vi "ReviewQnsPaper1(SubVI).vi"(11 "connection reference":T2) -> (0 "close?":bool, 3 "connection reference out":T2)   [LabVIEW 2013]
uses:
  <vilib>/addons/database/Connection.llb/Conn ObjectReference.ctl
  FYP_LabviewGlobal(SubVI).vi
  <vilib>/addons/database/_DB Variant To Data/Database Variant To Data.xnode
  <vilib>/addons/database/NI_Database_API.lvlib
panel:
  out "Choice":string
  out "Answer":string
  out "D":bool
  out "C":bool
  out "B":bool
  out "A":bool
  out "D":string
  out "C":string
  out "B":string
  out "A":string
  out "DInd":bool
  out "CInd":bool
  out "BInd":bool
  out "AInd":bool
  out "Question":string
  out "Why?":string
  in  "SelectQn":T1(radio)
  in  "Close":bool
  out "Marks%":dbl
  out "TotalMarks":string
  # "% )"
  # "Your Score is :"
  # "("
  # "Questions:"
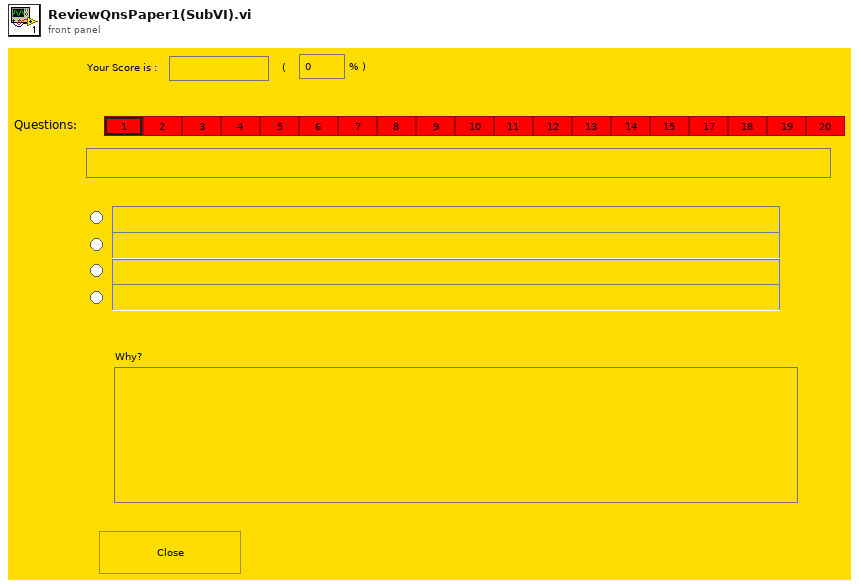
[diagram p1: front panel]
types:
  T1 = enum32{"1", "2", "3", "4", "5", "6", "7", "8", "9", "10", "11", "12", "13", "14", "15", "16", "17", "18", "19", "20"}
  T2 = typedef "NI_Database_API.lvlib/Conn ObjectReference.ctl" = refnum<k1>
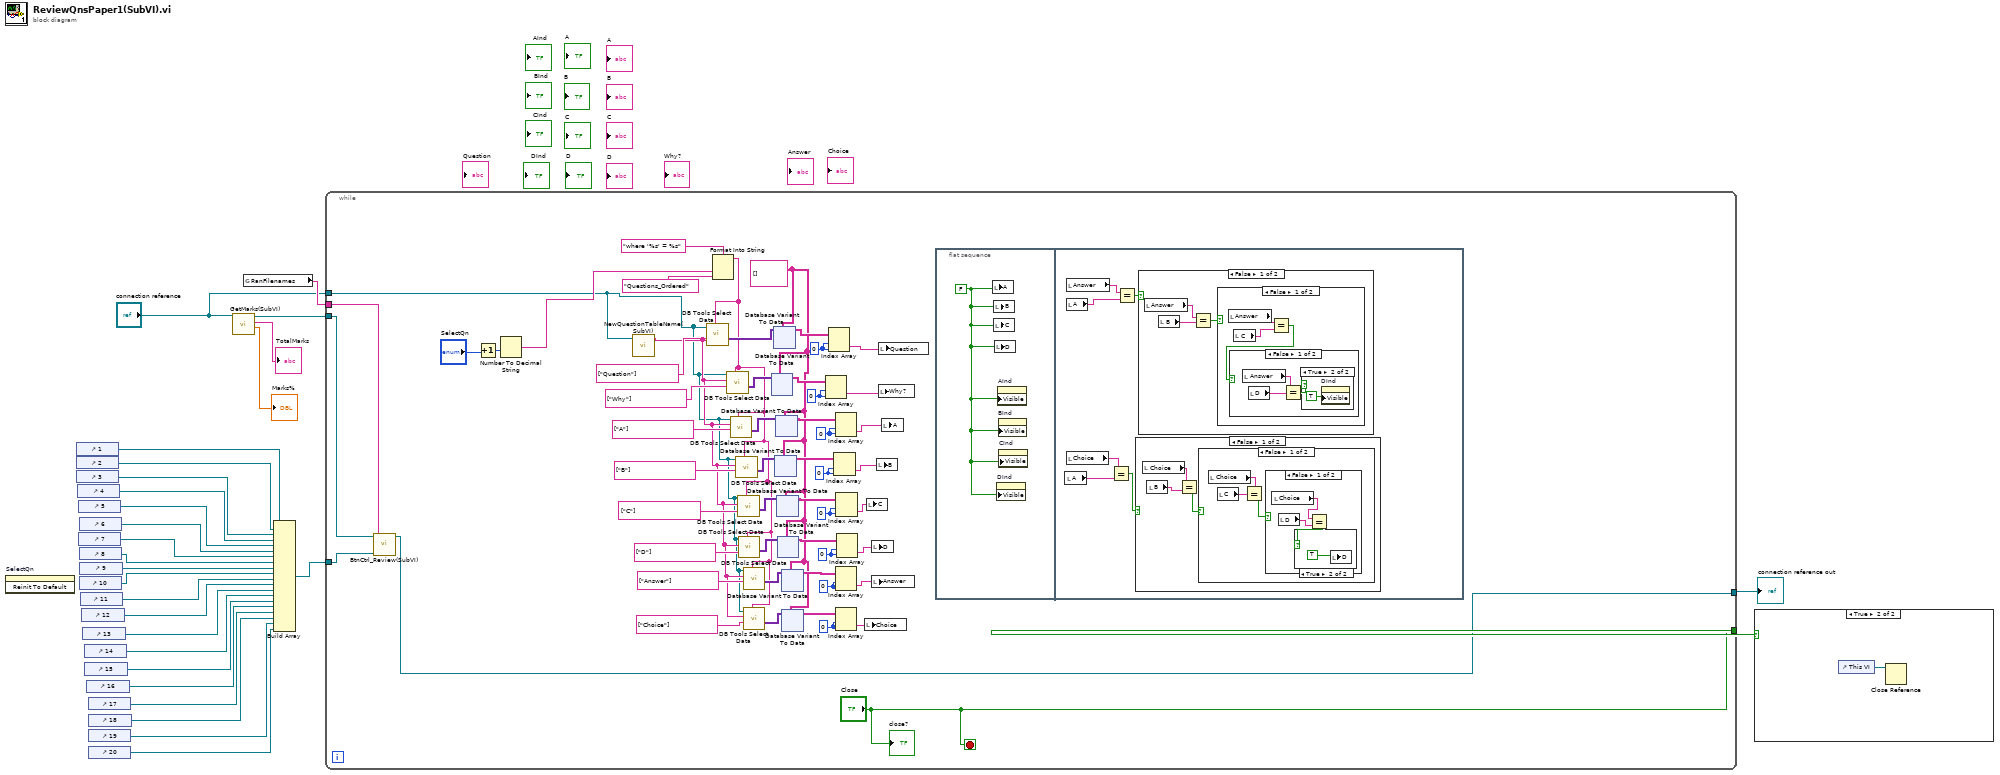
[diagram p0: block diagram]
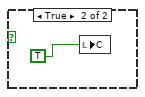
[diagram p4: hidden frame]
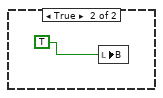
[diagram p5: hidden frame]
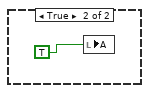
[diagram p6: hidden frame]
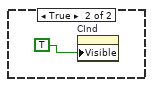
[diagram p8: hidden frame]
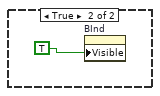
[diagram p9: hidden frame]
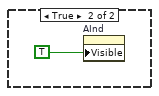
[diagram p10: hidden frame]
diagram:
  n1 = invoke on="SelectQn" class="RadioBtnsControl (strict)" method="Reinit To Default"() -> ()  [unwired: 3 in, 3 out]
  n2 = control-ref of="1"() -> (w21:refnum<vi>)
  n3 = control-ref of="2"() -> (w20:refnum<vi>)
  n4 = control-ref of="3"() -> (w19:refnum<vi>)
  n5 = control-ref of="4"() -> (w18:refnum<vi>)
  n6 = control-ref of="5"() -> (w17:refnum<vi>)
  n7 = control-ref of="7"() -> (w15:refnum<vi>)
  n8 = control-ref of="6"() -> (w16:refnum<vi>)
  n9 = control-ref of="8"() -> (w14:refnum<vi>)
  n10 = control-ref of="10"() -> (w12:refnum<vi>)
  n11 = control-ref of="9"() -> (w13:refnum<vi>)
  n12 = control-ref of="11"() -> (w11:refnum<vi>)
  n13 = control-ref of="12"() -> (w10:refnum<vi>)
  n14 = control-ref of="13"() -> (w9:refnum<vi>)
  n15 = control-ref of="14"() -> (w8:refnum<vi>)
  n16 = control-ref of="15"() -> (w7:refnum<vi>)
  n17 = control-ref of="16"() -> (w2:refnum<vi>)
  n18 = control-ref of="17"() -> (w3:refnum<vi>)
  n19 = control-ref of="19"() -> (w5:refnum<vi>)
  n20 = control-ref of="20"() -> (w6:refnum<vi>)
  n21 = control-ref of="18"() -> (w4:refnum<vi>)
  n22 = call "GetMarks(SubVI).vi"("connection reference 3"="connection reference") -> ("Marks%"=→"Marks%":dbl, "TotalMarks"=→"TotalMarks":string, "connection reference 2"=w25:T2)  [unwired: 8 in]
  n23 = global read "FYP_LabviewGlobal(SubVI).vi" "RanFilenames"() -> (w26:string[])
  n24 = Build Array(w21, w20, w19, w18, w17, w16, w15, w14, w13, w12, w11, w10, w9, w8, w7, w2, w3, w4, w5, w6) -> (w24:refnum<vi>[])
  n25 = while {
    tunnel: w26 -> [w80]
    tunnel: w25 -> [w81]
    tunnel: w24 -> [w79]
    tunnel: [w78] -> w23
    tunnel: ["Close"] -> w22
    tunnel: "connection reference" -> [w29]
    stop <- "Close" stop-if-true
    w38 = 0 ("disabled index (col)")
    w42 = 0 ("disabled index (col)")
    w47 = 0 ("disabled index (col)")
    w52 = 0 ("disabled index (col)")
    w56 = 0 ("disabled index (col)")
    w60 = 0 ("disabled index (col)")
    w65 = 0 ("disabled index (col)")
    w68 = 0 ("disabled index (col)")
    w35 = string[][] []
    n26 = call "BtnCtrl_Review(SubVI).vi"("ButtonControlArray"=w79, "RanFilenames"=w80, "connection reference"=w81) -> ("connection reference out"=w78:T2)  [unwired: 8 in]
    n27 = Increment(x="SelectQn") -> (x+1=w75:T1)
    n28 = Number To Decimal String(number=w75) -> (decimal integer string=w77:string)  [unwired: 1 in]
    n29 = call "NewQuestionTableName(SubVI).vi"("connection reference"=w29) -> ("String"=w30:string)  [unwired: 10 in]
    n30 = Format Into String(format string="where '%s' = %s", w77, "Questions_Ordered") -> (resulting string=w34:string)  [unwired: 2 in, 1 out]
    n31 = call <vilib>:"DB Tools Select Data.vi"("condition"=w34, "columns"=string[] ["Question"], "table"=w30, "connection reference"=w29) -> ("data"=w71:variant[][])  [unwired: 2 in, 2 out]
    n32 = call <vilib>:"DB Tools Select Data.vi"("condition"=w34, "columns"=string[] ["Why"], "table"=w30, "connection reference"=w29) -> ("data"=w64:variant[][])  [unwired: 2 in, 2 out]
    n33 = call <vilib>:"DB Tools Select Data.vi"("condition"=w34, "columns"=string[] ["A"], "table"=w30, "connection reference"=w29) -> ("data"=w61:variant[][])  [unwired: 2 in, 2 out]
    n34 = call <vilib>:"DB Tools Select Data.vi"("condition"=w34, "columns"=string[] ["B"], "table"=w30, "connection reference"=w29) -> ("data"=w54:variant[][])  [unwired: 2 in, 2 out]
    n35 = call <vilib>:"DB Tools Select Data.vi"("condition"=w34, "columns"=string[] ["C"], "table"=w30, "connection reference"=w29) -> ("data"=w50:variant[][])  [unwired: 2 in, 2 out]
    n36 = call <vilib>:"DB Tools Select Data.vi"("condition"=w34, "columns"=string[] ["D"], "table"=w30, "connection reference"=w29) -> ("data"=w45:variant[][])  [unwired: 2 in, 2 out]
    n37 = call <vilib>:"DB Tools Select Data.vi"("condition"=w34, "columns"=string[] ["Answer"], "table"=w30, "connection reference"=w29) -> ("data"=w40:variant[][])  [unwired: 2 in, 2 out]
    n38 = call <vilib>:"DB Tools Select Data.vi"("condition"=w34, "columns"=string[] ["Choice"], "table"=w30, "connection reference"=w29) -> ("data"=w36:variant[][])  [unwired: 2 in, 2 out]
    n39 = xnode "Database Variant To Data"("database variant"=w64, "type"=w35) -> ("data"=w66:string[][])  [unwired: 1 in, 1 out]
    n40 = xnode "Database Variant To Data"("database variant"=w71, "type"=w35) -> ("data"=w70:string[][])  [unwired: 1 in, 1 out]
    n41 = xnode "Database Variant To Data"("database variant"=w54, "type"=w35) -> ("data"=w55:string[][])  [unwired: 1 in, 1 out]
    n42 = xnode "Database Variant To Data"("database variant"=w61, "type"=w35) -> ("data"=w59:string[][])  [unwired: 1 in, 1 out]
    n43 = xnode "Database Variant To Data"("database variant"=w50, "type"=w35) -> ("data"=w51:string[][])  [unwired: 1 in, 1 out]
    n44 = xnode "Database Variant To Data"("database variant"=w45, "type"=w35) -> ("data"=w46:string[][])  [unwired: 1 in, 1 out]
    n45 = xnode "Database Variant To Data"("database variant"=w40, "type"=w35) -> ("data"=w41:string[][])  [unwired: 1 in, 1 out]
    n46 = xnode "Database Variant To Data"("database variant"=w36, "type"=w35) -> ("data"=w37:string[][])  [unwired: 1 in, 1 out]
    n47 = Index Array(array=w66, index (row)=w65, index (col)=w65) -> (element=w63:string)
    n48 = Index Array(array=w70, index (row)=w68, index (col)=w68) -> (element=w69:string)
    n49 = Index Array(array=w55, index (row)=w56, index (col)=w56) -> (element=w53:string)
    n50 = Index Array(array=w59, index (row)=w60, index (col)=w60) -> (element=w58:string)
    n51 = Index Array(array=w41, index (row)=w42, index (col)=w42) -> (element=w32:string)
    n52 = Index Array(array=w37, index (row)=w38, index (col)=w38) -> (element=w31:string)
    n53 = Index Array(array=w51, index (row)=w52, index (col)=w52) -> (element=w49:string)
    n54 = Index Array(array=w46, index (row)=w47, index (col)=w47) -> (element=w43:string)
    n55 = local write "Choice"(w31) -> ()
    n56 = local write "C"(w49) -> ()
    n57 = local write "D"(w43) -> ()
    n58 = local write "Answer"(w32) -> ()
    n59 = local write "B"(w53) -> ()
    n60 = local write "Why?"(w63) -> ()
    n61 = local write "Question"(w69) -> ()
    n62 = local write "A"(w58) -> ()
    n63 = flat-sequence {
      frame #0 {
        w171 = FALSE
        n64 = local write "A"(w171) -> ()
        n65 = local write "B"(w171) -> ()
        n66 = local write "C"(w171) -> ()
        n67 = local write "D"(w171) -> ()
        n68 = property on="DInd" class="Bool"("Visible"=w171) -> ()  [unwired: 2 in, 2 out]
        n69 = property on="AInd" class="Bool"("Visible"=w171) -> ()  [unwired: 2 in, 2 out]
        n70 = property on="BInd" class="Bool"("Visible"=w171) -> ()  [unwired: 2 in, 2 out]
        n71 = property on="CInd" class="Bool"("Visible"=w171) -> ()  [unwired: 2 in, 2 out]
      }
      frame #1 {
        n72 = local read "A"() -> (w173:string)
        n73 = local read "Answer"() -> (w177:string)
        n74 = local read "A"() -> (w176:string)
        n75 = local read "Choice"() -> (w174:string)
        n76 = Equal?(x=w174, y=w173) -> (x = y?=w172:bool)
        n77 = Equal?(x=w177, y=w176) -> (x = y?=w175:bool)
        n78 = case shown="False" w172 {
          frame False {
            n79 = local read "Choice"() -> (w180:string)
            n80 = local read "B"() -> (w179:string)
            n81 = Equal?(x=w180, y=w179) -> (x = y?=w178:bool)
            n82 = case shown="False" w178 {
              frame False {
                n83 = local read "Choice"() -> (w183:string)
                n84 = local read "C"() -> (w182:string)
                n85 = Equal?(x=w183, y=w182) -> (x = y?=w181:bool)
                n86 = case shown="False" w181 {
                  frame False {
                    n87 = local read "Choice"() -> (w186:string)
                    n88 = local read "D"() -> (w185:string)
                    n89 = Equal?(x=w186, y=w185) -> (x = y?=w184:bool)
                    n90 = case shown="True" w184 {
                      frame False {
                      }
                      frame True {
                        n91 = local write "D"(TRUE) -> ()
                      }
                    }
                  }
                  frame True {
                    n92 = local write "C"(TRUE) -> ()
                  }
                }
              }
              frame True {
                n93 = local write "B"(TRUE) -> ()
              }
            }
          }
          frame True {
            n94 = local write "A"(TRUE) -> ()
          }
        }
        n95 = case shown="False" w175 {
          frame False {
            n96 = local read "Answer"() -> (w193:string)
            n97 = local read "B"() -> (w192:string)
            n98 = Equal?(x=w193, y=w192) -> (x = y?=w191:bool)
            n99 = case shown="False" w191 {
              frame False {
                n100 = local read "Answer"() -> (w196:string)
                n101 = local read "C"() -> (w195:string)
                n102 = Equal?(x=w196, y=w195) -> (x = y?=w194:bool)
                n103 = case shown="False" w194 {
                  frame False {
                    n104 = local read "Answer"() -> (w199:string)
                    n105 = local read "D"() -> (w198:string)
                    n106 = Equal?(x=w199, y=w198) -> (x = y?=w197:bool)
                    n107 = case shown="True" w197 {
                      frame False {
                      }
                      frame True {
                        n108 = property on="DInd" class="Bool"("Visible"=TRUE) -> ()  [unwired: 2 in, 2 out]
                      }
                    }
                  }
                  frame True {
                    n109 = property on="CInd" class="Bool"("Visible"=TRUE) -> ()  [unwired: 2 in, 2 out]
                  }
                }
              }
              frame True {
                n110 = property on="BInd" class="Bool"("Visible"=TRUE) -> ()  [unwired: 2 in, 2 out]
              }
            }
          }
          frame True {
            n111 = property on="AInd" class="Bool"("Visible"=TRUE) -> ()  [unwired: 2 in, 2 out]
          }
        }
      }
    }
    "close?" <- "Close"
  }
  "connection reference out" <- w23
  n112 = case shown="True" w22 {
    frame False {
    }
    frame True {
      n113 = control-ref of="This VI"() -> (w468:refnum<vi>)
      n114 = Close Reference(reference=w468) -> ()  [unwired: 1 in, 1 out]
    }
  }
